vi "Encoder.vi"() -> ()   [LabVIEW 2021]
panel:
  out "Y 0":bool
  out "Y 2":bool
  out "Y 1":bool
  in  "x 1":bool
  in  "x 7":bool
  in  "x 6":bool
  in  "x 5":bool
  in  "x 4":bool
  in  "x 3":bool
  in  "x 2":bool
  in  "x 0":bool
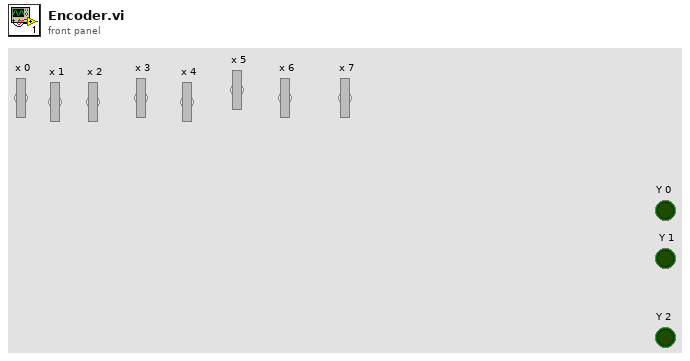
[diagram p1: front panel]
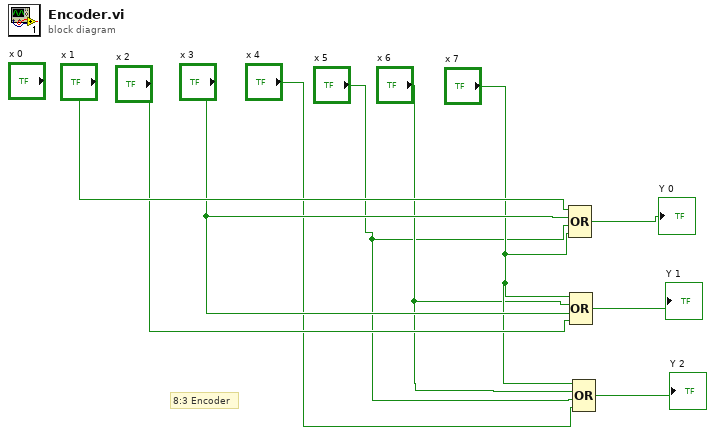
[diagram p0: block diagram]
diagram:
  # "8:3 Encoder"
  n1 = Compound Arithmetic op=OR("x 1", "x 3", "x 5", "x 7") -> (→"Y 0":bool)
  n2 = Compound Arithmetic op=OR("x 7", "x 6", "x 3", "x 2") -> (→"Y 1":bool)
  n3 = Compound Arithmetic op=OR("x 7", "x 6", "x 5", "x 4") -> (→"Y 2":bool)
